vi "Add Malleable VI in Logic.vi"(0 "Logic VI":refnum<vi>, 5 "SubVIs Ref":refnum<vi>[](array[refnum]), 11 "error in (no error)":errorcluster) -> (15 "error out":errorcluster)   [LabVIEW 2021, in "Migrator.lvlib"]
uses:
  Migrator.lvlib
  <vilib>/Utility/miscctls.llb/LVPointTypeDef.ctl
  <vilib>/ErrorRing/Error Ring.xnode
  Migrator Reusables/Migrator Reusables.lvlib
  Path Functions/Path Functions.lvlib
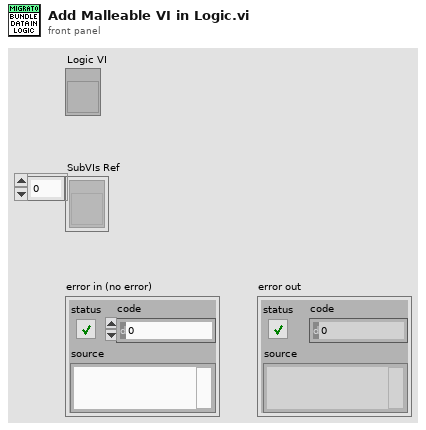
[diagram p1: front panel]
types:
  T1 = typedef "LVPointTypeDef.ctl" = cluster{"Horizontal":i16, "Vertical":i16}
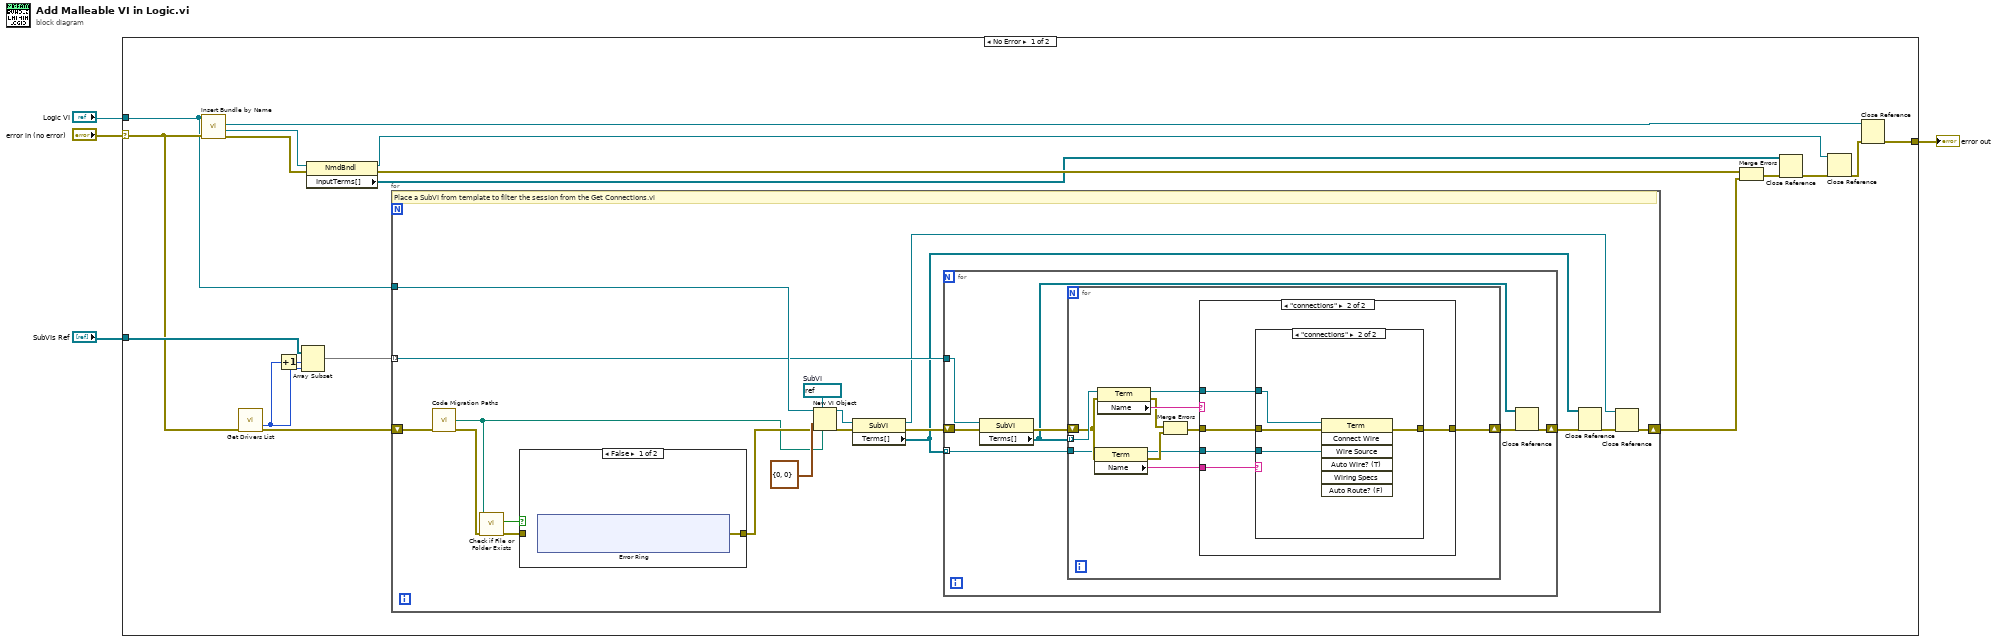
[diagram p0: block diagram]
diagram:
  n1 = case shown="No Error" "error in (no error)" {
    selector: "error in (no error)" -> [w12 w73]
    tunnel: [w22 w73] -> w4
    tunnel: "SubVIs Ref" -> [w13 _]
    tunnel: "Logic VI" -> [w8 _]
    frame No Error {
      n2 = call "Insert Bundle by Name.vi"("error in (no error)"=w12, "VI in"=w8) -> ("error out"=w16:errorcluster, "Named Bundler"=w19:refnum<vi>, "Wrapper Refnum"=w21:refnum<vi>)  [unwired: 7 in]
      n3 = call "Get Drivers List.vi"("error in (no error)"=w12) -> ("Removed Duplicates Size"=w6:i32, "error out"=w9:errorcluster)  [unwired: 9 in, 4 out]
      n4 = Increment(x=w6) -> (x+1=w5:i32)
      n5 = Array Subset(array=w13, index=w5, length=w6) -> (w10:refnum<vi>[])
      n6 = property class="NmdBndl"(reference=w19, error in=w16) -> (reference out=w14:refnum<vi>, error out=w15:errorcluster, "InputTerms[]"=w11:refnum<vi>[])
      n7 = for {
        tunnel: w10 -> [w35] mode=indexing
        tunnel: w8 -> [w38]
        shift-right: [w30] -> w7
        shift-left: w9 -> [w40]
        w39 = refnum<vi> refnum  # SubVI
        # "Place a SubVI from template to filter the session from the Get Connections.vi"
        n8 = call "Code Migration Paths.vi"("error in (no error)"=w40) -> ("Get Resource VI"=w23:path, "error out"=w25:errorcluster)  [unwired: 6 in, 7 out]
        n9 = call <vilib>:"Check if File or Folder Exists.vi"("error in (no error)"=w25, "path"=w23) -> ("error out"=w26:errorcluster, "file or folder exists?"=w27:bool)  [unwired: 7 in, 1 out]
        n10 = case shown="False" w27 {
          tunnel: w26 -> [_ w43]
          tunnel: [w41 w43] -> w24
          frame False {
            n11 = xnode "Error Ring"() -> ("error out"=w41:errorcluster)
          }
          frame True {
          }
        }
        n12 = New VI Object(vi object class=w39, owner refnum=w38, position/next to=T1 {"Horizontal"=0, "Vertical"=0} ("location"), 6:w23, 8:w24) -> (object refnum=w31:refnum<vi>, 0:w37:errorcluster)  [unwired: 3 in]
        n13 = property class="SubVI"(reference=w31, error in=w37) -> (reference out=w28:refnum<vi>, error out=w36:errorcluster, "Terms[]"=w33:refnum<vi>[])
        n14 = for {
          tunnel: w33 -> [w47] mode=indexing
          tunnel: w35 -> [w50]
          shift-right: [w44] -> w34
          shift-left: w36 -> [w49]
          n15 = property class="SubVI"(reference=w50, error in=w49) -> (error out=w48:errorcluster, "Terms[]"=w45:refnum<vi>[])  [unwired: 1 out]
          n16 = for {
            tunnel: w45 -> [w61] mode=indexing
            tunnel: w47 -> [w59]
            shift-right: [w51] -> w46
            shift-left: w48 -> [w60]
            n17 = property class="Term"(reference=w59, error in=w60) -> (reference out=w52:refnum<vi>, error out=w55:errorcluster, "Name"=w57:string)
            n18 = property class="Term"(reference=w61, error in=w60) -> (reference out=w53:refnum<vi>, error out=w56:errorcluster, "Name"=w58:string)
            n19 = Merge Errors(w56, w55) -> (w54:errorcluster)
            n20 = case shown="\"connections\"" w58 {
              tunnel: w57 -> [_ w67]
              tunnel: w54 -> [w62 w65]
              tunnel: w53 -> [_ w66]
              tunnel: w52 -> [_ w64]
              tunnel: [w62 w63] -> w51
              frame Default {
              }
              frame "connections" {
                n21 = case shown="\"connections\"" w67 {
                  tunnel: w66 -> [_ w72]
                  tunnel: w65 -> [w68 w71]
                  tunnel: w64 -> [_ w70]
                  tunnel: [w68 w69] -> w63
                  frame Default {
                  }
                  frame "connections" {
                    n22 = invoke class="Term" method="Connect Wire"(reference=w72, error in=w71, "Wire Source"=w70) -> (error out=w69:errorcluster)  [unwired: 4 in, 6 out]
                  }
                }
              }
            }
          }
          n23 = Close Reference(reference=w45, error in (no error)=w46) -> (error out=w44:errorcluster)
        }
        n24 = Close Reference(reference=w33, error in (no error)=w34) -> (error out=w32:errorcluster)
        n25 = Close Reference(reference=w28, error in (no error)=w32) -> (error out=w30:errorcluster)
      }
      n26 = Merge Errors(w15, w7) -> (w18:errorcluster)
      n27 = Close Reference(reference=w11, error in (no error)=w18) -> (error out=w17:errorcluster)
      n28 = Close Reference(reference=w14, error in (no error)=w17) -> (error out=w20:errorcluster)
      n29 = Close Reference(reference=w21, error in (no error)=w20) -> (error out=w22:errorcluster)
    }
    frame Error {
    }
  }
  "error out" <- w4
